vi "Get CalPoints.vi"() -> ()   [LabVIEW 2015, in "ECS-RT.lvlib"]
uses:
  ECS-RT.lvlib
  <vilib>/addons/Software Calibration Management/_CalPointResources/SCM - RT Types.ctl
  Globals/Calpoint IDs.vi
  <vilib>/addons/Software Calibration Management/_CalPointResources/scm32.dll
panel:
  out "Get Cal Exec":dbl caption="[msec]"
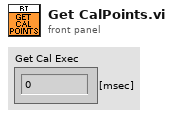
[diagram p1: front panel]
types:
  T1 = typedef "SCM - RT Types.ctl" = enum32{"U8", "U32", "I8", "I32", "SGL", "TBL1D_SGL", "TBL2D_SGL", "U32_ENUM", "BOOL", "Array1D_SGL", "Array2D_SGL", "STR"}
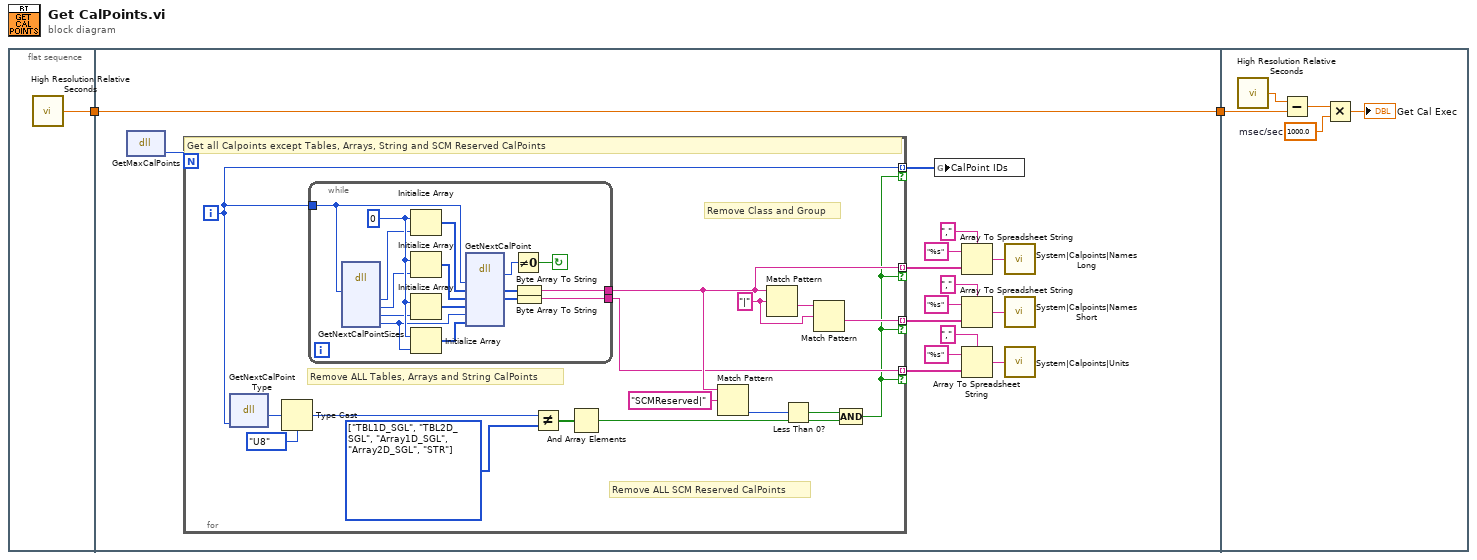
[diagram p0: block diagram]
diagram:
  n1 = flat-sequence {
    tunnel: [w3] -> w2
    tunnel: w2 -> [w17]
    tunnel: [w17] -> w1
    tunnel: w1 -> [w54]
    frame #0 {
      n2 = call <vilib>:"High Resolution Relative Seconds.vi"() -> ("relative seconds"=w3:dbl)
    }
    frame #1 {
      n3 = dll-call lib="C:/Program Files (x86)/National Instruments/LabVIEW 2015/vi.lib/addons/Software Calibration Management/_CalPointResources/scm*.*" fn="GetMaxCalPoints"() -> ("NumCalPoints"=w18:i32)  [unwired: 3 in, 2 out]
      n4 = for {
        N: w18 -> [_]
        tunnel: [w24] -> w12 mode=indexing if=w19
        tunnel: [w32] -> w16 mode=indexing if=w19
        tunnel: [w21] -> w8 mode=indexing if=w19
        tunnel: [w20] -> w4 mode=indexing if=w19
        i -> [w32]
        w23 = "|" ("regular expression")
        w29 = T1[] [enum."TBL1D_SGL", enum."TBL2D_SGL", enum."Array1D_SGL", enum."Array2D_SGL", enum."STR"] items=["U8", "U32", "I8", "I32", "SGL", "TBL1D_SGL", "TBL2D_SGL", "U32_ENUM", "BOOL", "Array1D_SGL", "Array2D_SGL", "STR"]
        # "Remove ALL Tables, Arrays and String CalPoints"
        # "Remove ALL SCM Reserved CalPoints"
        # "Remove Class and Group"
        # "Get all Calpoints except Tables, Arrays, String and SCM Reserved CalPoints"
        n5 = dll-call lib="C:/Program Files (x86)/National Instruments/LabVIEW 2015/vi.lib/addons/Software Calibration Management/_CalPointResources/scm*.*" fn="GetNextCalPointType"("ID"=w32) -> ("Type"=w33:u32)  [unwired: 4 in, 2 out]
        n6 = Type Cast(type=SCM_-_RT_Types."U8" ("SCM Types"), x=w33) -> (*(type *) &x=w31:T1)
        n7 = while {
          tunnel: [w50] -> w21
          tunnel: w32 -> [w37]
          tunnel: [w35] -> w20
          stop <- w38 continue-if-true
          w49 = u8 0
          n8 = dll-call lib="C:/Program Files (x86)/National Instruments/LabVIEW 2015/vi.lib/addons/Software Calibration Management/_CalPointResources/scm*.*" fn="GetNextCalPointSizes"("ID"=w37) -> ("ClassGroupName"=w44:i32, "Units"=w43:i32, "Description"=w42:i32, "Data"=w40:i32)  [unwired: 4 in, 7 out]
          n9 = Initialize Array(w49, w44) -> (w48:u8[])
          n10 = Initialize Array(w49, w43) -> (w47:u8[])
          n11 = Initialize Array(w49, w42) -> (w46:u8[])
          n12 = Initialize Array(w49, w40) -> (w45:u8[])
          n13 = dll-call lib="C:/Program Files (x86)/National Instruments/LabVIEW 2015/vi.lib/addons/Software Calibration Management/_CalPointResources/scm*.*" fn="GetNextCalPoint"("ID"=w37, "ClassGroupName"=w48, "Units"=w47, "Description"=w46, "DataSize"=w40, "Data"=w45) -> ("Error"=w39:i32, "ClassGroupName"=w41:u8[], "Units"=w36:u8[])  [unwired: 7 in, 2 out]
          n14 = Not Equal To 0?(x=w39) -> (x != 0?=w38:bool)
          n15 = Byte Array To String(unsigned byte array=w41) -> (string=w50:string)
          n16 = Byte Array To String(unsigned byte array=w36) -> (string=w35:string)
        }
        n17 = Not Equal?(x=w31, y=w29) -> (x != y?=w30:bool[])
        n18 = And Array Elements(Boolean array=w30) -> (logical AND=w25:bool)
        n19 = Match Pattern(string=w21, regular expression="SCMReserved|" ("string")) -> (offset past match=w28:i32)  [unwired: 1 in, 3 out]
        n20 = Match Pattern(string=w21, regular expression=w23) -> (after substring=w22:string)  [unwired: 1 in, 3 out]
        n21 = Less Than 0?(x=w28) -> (x < 0?=w26:bool)
        n22 = Match Pattern(string=w22, regular expression=w23) -> (after substring=w24:string)  [unwired: 1 in, 3 out]
        n23 = Compound Arithmetic op=AND(w26, w25) -> (w19:bool)
      }
      n24 = global write "Calpoint IDs.vi" "CalPoint IDs"(w16) -> ()
      n25 = Array To Spreadsheet String(delimiter (Tab)=",", array=w8, 3:"%s" ("format string")) -> (spreadsheet string=w11:string)
      n26 = Array To Spreadsheet String(delimiter (Tab)=",", array=w12, 3:"%s" ("format string")) -> (spreadsheet string=w13:string)
      n27 = Array To Spreadsheet String(delimiter (Tab)=",", array=w4, 3:"%s" ("format string")) -> (spreadsheet string=w7:string)
      n28 = call "System|Calpoints|NamesLong"("Value"=w11) -> ()
      n29 = call "System|Calpoints|NamesShort"("Value"=w13) -> ()
      n30 = call "System|Calpoints|Units"("Value"=w7) -> ()
    }
    frame #2 {
      w52 = 1000.0  # msec/sec
      n31 = call <vilib>:"High Resolution Relative Seconds.vi"() -> ("relative seconds"=w55:dbl)
      n32 = Subtract(x=w55, y=w54) -> (x-y=w53:dbl)
      n33 = Multiply(x=w53, y=w52) -> (x*y=→"Get Cal Exec":dbl)
    }
  }
